vi "CloneMethod.vi"(0 "ClassWriter.lvclass":refnum<class "ClassWriter.lvclass">, 1 "VIItemRefIn":refnum<vi>, 2 "NewVIPath":path, 3 "LibraryOwners":refnum<vi>[](array[refnum]), 4 "OpenVIWhenDone":bool, 5 "error in (no error)":errorcluster, 7 "ViDescription":string) -> (14 "ClassWriter.lvclass":refnum<class "ClassWriter.lvclass">, 19 "error out":errorcluster)   [LabVIEW 2020, in "ClassWriter.lvclass"]
uses:
  <resource>/Framework/Providers/Open_GDS/ClassProviders/Provider_BaseClassInterface/ClassWriter_class/ClassWriter.lvclass
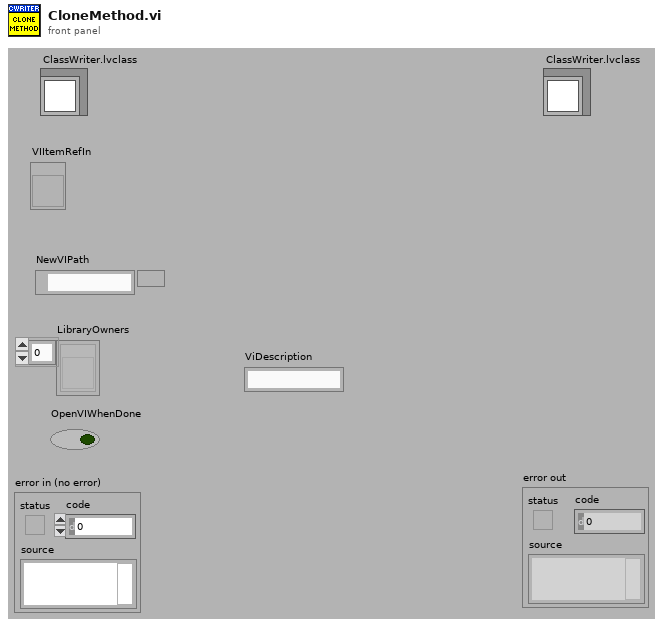
[diagram p1: front panel]
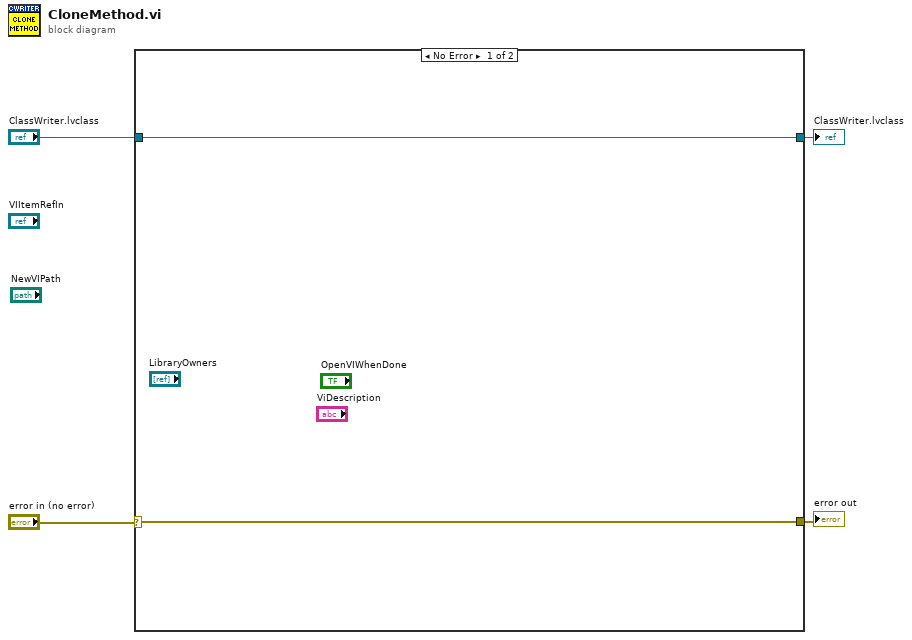
[diagram p0: block diagram]
diagram:
  n1 = case shown="No Error" "error in (no error)" {
    selector: "error in (no error)" -> [w5 w7]
    tunnel: "ClassWriter.lvclass" -> [w6 w8]
    tunnel: [w5 w7] -> w3
    tunnel: [w6 w8] -> w2
    frame No Error {
    }
    frame Error {
    }
  }
  "ClassWriter.lvclass" <- w2
  "error out" <- w3
